vi "XML to Set Points.vi"(0 "XML Data":string) -> ()   [LabVIEW 2013]
uses:
  Types/Set Points.ctl
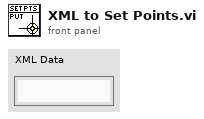
[diagram p1: front panel]
types:
  T1 = typedef "Set Points.ctl" = cluster{"X Position Set-point":dbl, "Y Position Set-point":dbl, "Z Position Set-point":dbl, "Z Scan Set-point":dbl, "Version":string}
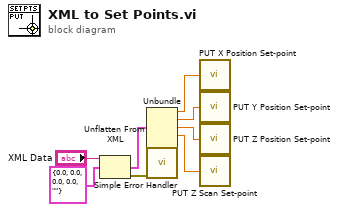
[diagram p0: block diagram]
diagram:
  n1 = Unflatten From XML(xml string="XML Data", type=T1 {"X Position Set-point"=0.0, "Y Position Set-point"=0.0, "Z Position Set-point"=0.0, "Z Scan Set-point"=0.0, "Version"=""} ("Set Points")) -> (value=w5:T1, error out=w8:errorcluster)  [unwired: 1 in]
  n2 = Unbundle(w5) -> ("X Position Set-point"=w2:dbl, "Y Position Set-point"=w4:dbl, "Z Position Set-point"=w3:dbl, "Z Scan Set-point"=w1:dbl)  [unwired: 1 out]
  n3 = call <vilib>:"Simple Error Handler.vi"("error in (no error)"=w8) -> ()  [unwired: 4 in, 5 out]
  n4 = call "PUT X Position Set-point.vi"("X Position Set-point"=w2) -> ()
  n5 = call "PUT Y Position Set-point.vi"("Y Position Set-point"=w4) -> ()
  n6 = call "PUT Z Position Set-point.vi"("Z Position Set-point"=w3) -> ()
  n7 = call "PUT Z Scan Set-point.vi"("Z Scan Set-point"=w1) -> ()
